vi "Init.vi"(8 "error in (no error)":errorcluster, 10 "Intrs Configs":T1, 11 "IMSS Remote Actor in":refnum<class "IMSS Remote Actor.lvclass">) -> (0 "error out":errorcluster, 3 "IMSS Remote Actor out":refnum<class "IMSS Remote Actor.lvclass">)   [LabVIEW 2023, in "MSS Remote Actor - Interface.lvlib" / "IMSS Remote Actor.lvclass"]
uses:
  IMSS Remote Actor.lvclass
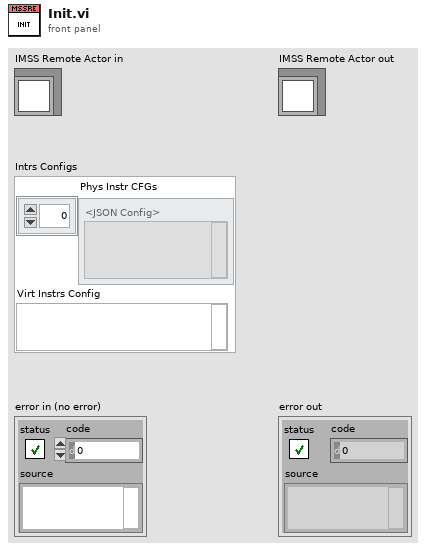
[diagram p1: front panel]
types:
  T1 = cluster{"Phys Instr CFGs":string[], "Virt Instrs Config":string}
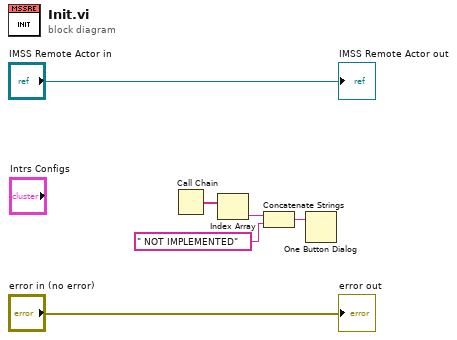
[diagram p0: block diagram]
diagram:
  n1 = Call Chain() -> (call chain=w4:string[])
  n2 = Index Array(array=w4) -> (element=w2:string)  [unwired: 1 in]
  n3 = Concatenate Strings(w2, " NOT IMPLEMENTED" ("string")) -> (w3:string)
  n4 = One Button Dialog(message=w3) -> ()  [unwired: 1 in, 1 out]
  "error out" <- "error in (no error)"
  "IMSS Remote Actor out" <- "IMSS Remote Actor in"
